vi "Polyphase Filter (2D, SGL).vi"(6 "zero phase? (T)":bool=TRUE, 7 "init? (F)":bool, 8 "error in (no error)":errorcluster, 9 "factor":T1={"interpolation"=1, "decimation"=1}, 10 "FIR Coefficients":sgl[](array[numeric]), 11 "X":sgl[][](array[numeric])) -> (0 "error out":errorcluster, 3 "Filtered X":sgl[][](array[numeric]))   [LabVIEW 2020, in "NI_AAL_Filter.lvlib"]
doc: "Filters a signal continuously with a multirate filter."
uses:
  <vilib>/Analysis/NI_AAL_Filter.lvlib
  <vilib>/Analysis/3filter.llb/Polyphase Filter_Factor.ctl
  <vilib>/Analysis/NI_AALPro.lvlib
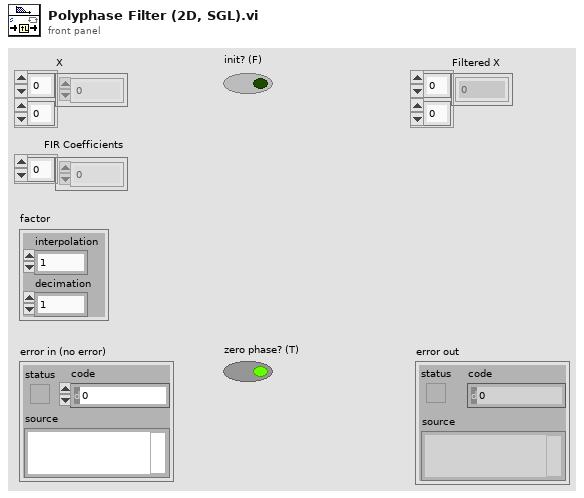
[diagram p1: front panel]
types:
  T1 = typedef "NI_AAL_Filter.lvlib/Polyphase Filter_Factor.ctl" = cluster{"interpolation":i32, "decimation":i32}
  T2 = typedef "NI_AAL_Filter.lvlib/Polyphase Filter_Mode.ctl" = i32
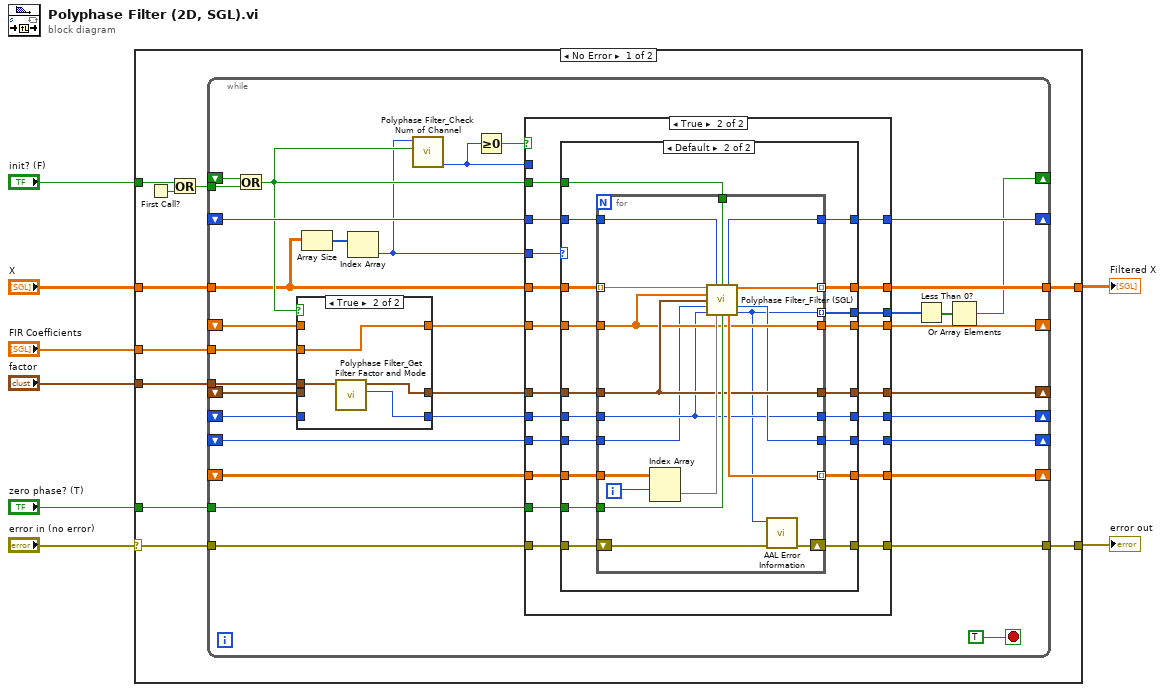
[diagram p0: block diagram]
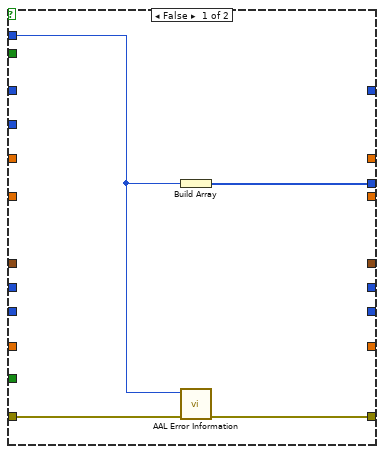
[diagram p2: hidden frame]
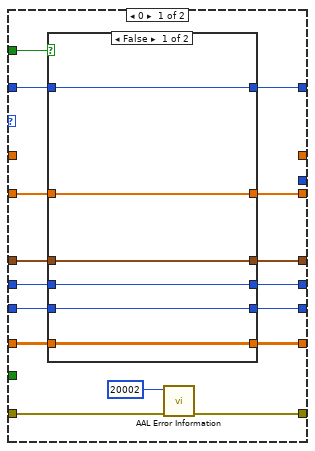
[diagram p3: hidden frame]
diagram:
  n1 = case shown="No Error" "error in (no error)" {
    selector: "error in (no error)" -> [w17 w145]
    tunnel: "factor" -> [w18 _]
    tunnel: "FIR Coefficients" -> [w16 _]
    tunnel: "X" -> [w15 _]
    tunnel: [w11 w145] -> w5
    tunnel: "init? (F)" -> [w13 _]
    tunnel: [w10 _] -> w2
    tunnel: "zero phase? (T)" -> [w9 _]
    frame No Error {
      n2 = First Call?() -> (First Call?: T/F=w14:bool)
      n3 = Or(x=w13, y=w14) -> (x .or. y?=w12:bool)
      n4 = while {
        tunnel: w18 -> [w49]
        tunnel: w16 -> [w50]
        tunnel: w12 -> [w36]
        shift-right: [w39] -> _
        shift-left: _ -> [w40]
        shift-right: [w23] -> _
        shift-left: _ -> [w27]
        shift-right: [w37] -> _
        shift-left: _ -> [w41]
        shift-right: [w28] -> _
        shift-left: _ -> [w47]
        shift-right: [w29] -> _
        shift-left: _ -> [w48]
        shift-right: [w30] -> _
        shift-left: _ -> [w46]
        tunnel: w9 -> [w35]
        shift-right: [w33] -> _
        shift-left: _ -> [w34]
        tunnel: w15 -> [w25]
        tunnel: [w42] -> w10
        tunnel: w17 -> [w22]
        tunnel: [w38] -> w11
        stop <- TRUE stop-if-true
        n5 = Or(x=w27, y=w36) -> (x .or. y?=w32:bool)
        n6 = case shown="True" w32 {
          tunnel: w49 -> [_ w144]
          tunnel: [w138 w143] -> w45
          tunnel: w50 -> [_ w143]
          tunnel: [w139 w142] -> w44
          tunnel: w48 -> [w139 _]
          tunnel: w47 -> [w138 _]
          tunnel: [w140 w141] -> w43
          tunnel: w46 -> [w140 _]
          frame False {
          }
          frame True {
            n7 = call <vilib>:"Polyphase Filter_Get Filter Factor and Mode.vi"("factor in"=w144) -> ("mode"=w141:T2, "factor out"=w142:T1)  [unwired: 9 in]
          }
        }
        n8 = Array Size(array=w25) -> (size(s)=w26:i32[])
        n9 = Index Array(array=w26) -> (element=w24:i32)  [unwired: 1 in]
        n10 = call <vilib>:"Polyphase Filter_Check Num of Channel.vi"("init"=w32, "number of channel"=w24) -> ("error"=w20:i32)  [unwired: 9 in]
        n11 = Greater Or Equal To 0?(x=w20) -> (x >= 0?=w21:bool)
        n12 = case shown="True" w21 {
          tunnel: w45 -> [_ w75]
          tunnel: w44 -> [_ w74]
          tunnel: w43 -> [_ w73]
          tunnel: [_ w72] -> w42
          tunnel: w41 -> [_ w71]
          tunnel: w40 -> [_ w70]
          tunnel: [_ w69] -> w39
          tunnel: [w55 w56] -> w19
          tunnel: [w54 w68] -> w38
          tunnel: [_ w67] -> w37
          tunnel: w35 -> [_ w66]
          tunnel: w34 -> [_ w65]
          tunnel: [_ w64] -> w33
          tunnel: w25 -> [_ w63]
          tunnel: w32 -> [_ w62]
          tunnel: [_ w61] -> w30
          tunnel: [_ w60] -> w29
          tunnel: [_ w59] -> w28
          tunnel: w24 -> [_ w58]
          tunnel: w22 -> [w53 w57]
          tunnel: w20 -> [w52 _]
          frame False {
            n13 = Build Array(w52) -> (w55:i32[])
            n14 = call <vilib>:"AAL Error Information.vi"("error in (no error)"=w53, "error code"=w52) -> ("error out"=w54:errorcluster)  [unwired: 9 in]
          }
          frame True {
            n15 = case shown="Default" w58 {
              tunnel: w75 -> [w80 w119]
              tunnel: w74 -> [w82 w118]
              tunnel: w73 -> [w84 w117]
              tunnel: [_ w116] -> w72
              tunnel: w71 -> [w89 w115]
              tunnel: w70 -> [w91 w114]
              tunnel: [w88 w113] -> w69
              tunnel: [_ w112] -> w56
              tunnel: w63 -> [_ w111]
              tunnel: [w77 w110] -> w68
              tunnel: w57 -> [w78 w109]
              tunnel: [w90 w108] -> w67
              tunnel: w62 -> [w87 w107]
              tunnel: w66 -> [_ w106]
              tunnel: w65 -> [w86 w105]
              tunnel: [w85 w104] -> w64
              tunnel: [w83 w103] -> w61
              tunnel: [w81 w102] -> w60
              tunnel: [w79 w101] -> w59
              frame 0 {
                n16 = case shown="False" w87 {
                  tunnel: [w97 _] -> w88
                  tunnel: w91 -> [w97 _]
                  tunnel: [w96 _] -> w90
                  tunnel: w89 -> [w96 _]
                  tunnel: [w95 _] -> w85
                  tunnel: w86 -> [w95 _]
                  tunnel: [w94 w100] -> w83
                  tunnel: w84 -> [w94 w100]
                  tunnel: w82 -> [w93 w99]
                  tunnel: [w93 w99] -> w81
                  tunnel: [w92 w98] -> w79
                  tunnel: w80 -> [w92 w98]
                  frame False {
                  }
                  frame True {
                  }
                }
                n17 = call <vilib>:"AAL Error Information.vi"("error in (no error)"=w78, "error code"=20002) -> ("error out"=w77:errorcluster)  [unwired: 9 in]
              }
              frame Default {
                n18 = for {
                  tunnel: w111 -> [w137] mode=indexing
                  tunnel: w119 -> [w124]
                  tunnel: w118 -> [w125]
                  tunnel: w117 -> [w122]
                  tunnel: [w136] -> w116 mode=indexing
                  tunnel: [w120] -> w112 mode=indexing
                  shift-right: [w133] -> w110
                  shift-left: w109 -> [w132]
                  tunnel: w114 -> [w121]
                  tunnel: [w123] -> w113
                  tunnel: w115 -> [w135]
                  tunnel: [w131] -> w108 mode=indexing
                  tunnel: w107 -> [w130]
                  tunnel: w106 -> [w129]
                  tunnel: w105 -> [w126]
                  tunnel: [w127] -> w104
                  tunnel: [w122] -> w103
                  tunnel: [w125] -> w102
                  tunnel: [w124] -> w101
                  i -> [w128]
                  n19 = Index Array(array=w135, index (row)=w128) -> (element=w134:sgl[])  [unwired: 1 in]
                  n20 = call <vilib>:"Polyphase Filter_Filter (SGL).vi"("X"=w137, "output phase in"=w126, "init? (F)"=w130, "FIR Coefficients"=w124, "factor"=w125, "skip point in"=w121, "mode"=w122, "State in"=w134, "zero phase? (T)"=w129) -> ("output phase out"=w127:i32, "Filtered X"=w136:sgl[], "skip point out"=w123:i32, "State out"=w131:sgl[], "error"=w120:i32)  [unwired: 2 in]
                  n21 = call <vilib>:"AAL Error Information.vi"("error in (no error)"=w132, "error code"=w120) -> ("error out"=w133:errorcluster)  [unwired: 9 in]
                }
              }
            }
          }
        }
        n22 = Less Than 0?(x=w19) -> (x < 0?=w31:bool[])
        n23 = Or Array Elements(Boolean array=w31) -> (logical OR=w23:bool)
      }
    }
    frame Error {
    }
  }
  "error out" <- w5
  "Filtered X" <- w2
